vi "GetTimeOnly.vi"(3 "Time Stamp":timestamp) -> (1 "Numeric":dbl)   [LabVIEW 2017]
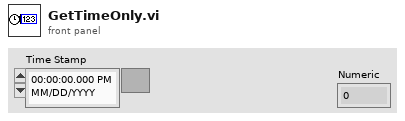
[diagram p1: front panel]
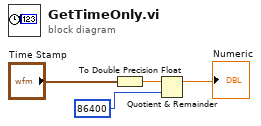
[diagram p0: block diagram]
diagram:
  n1 = To Double Precision Float(number="Time Stamp") -> (double precision float=w4:dbl)
  n2 = Quotient & Remainder(x=w4, y=86400) -> (x-y*floor(x/y)=→"Numeric":dbl)  [unwired: 1 out]
